vi "TOOLweb Spektren Pfad pruefen.vi"(6 "Aktionen":T3, 10 "labBaseName - SOLL":T1 caption="(82) labBaseName", 11 "Pfad Spektren - SOLL":T2 caption="Pfad Spektren") -> (2 "labBaseName - SOLL":T1 caption="(82) labBaseName", 3 "Pfad Spektren - SOLL":T2 caption="Pfad Spektren")   [LabVIEW 2020, in "FT-IR.lvlib" / "TOOLweb Interface.lvlib"]
doc: "Holt mit einer HTTP-POST-Anforderung gemäß TOOLweb-Protokoll Messdaten, Einstellungen und Diagnose-Information vom MKS MultiGas 2030 Analyzer. Alle Daten werden zeitsparend in einem einzigen Poll Request zusammengefasst, damit nur einmal eine TCP/IP-Verbindung geöffnet werden muss.\n\nAlle Ergebnis-Datentypen sind als Typdefinitionen in der Bibliothek \"Datentypen\" enthalten\" und erlauben so eine spätere Erweiterung.\n\nFalls \"Anzahl Gase\" unverbunden bleibt, wird der Standardwert 18 verwendet.\n \nFalls der TOOLWeb-Server nicht auf demselben Rechner arbeitet, kann mit \"IP-Adresse\" eine beliebiger Host adressiert werden. Ein unverbundener Eingang spricht den lokalen Host an."
uses:
  TOOLweb Interface.lvlib
  Spekten Pfad pruefen Aktionen.ctl
  Visualisierungs Elemente/Pfad-Eingabefeld.ctl
  Visualisierungs Elemente/String - Eingabefeld.ctl
  FGV FT-IR Aktionen.ctl
  FT-IR.lvlib
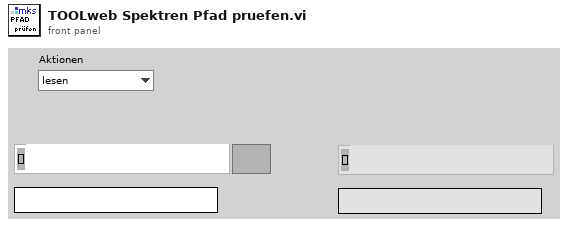
[diagram p1: front panel]
types:
  T1 = typedef "String - Eingabefeld.ctl" = string
  T2 = typedef "Pfad-Eingabefeld.ctl" = path
  T3 = typedef "FT-IR.lvlib/TOOLweb Interface.lvlib/Spekten Pfad pruefen Aktionen.ctl" = enum16{"lesen", "init", "prüfen", "setzen"}
  T4 = typedef "FT-IR.lvlib/FGV FT-IR Aktionen.ctl" = enum16{"lesen", "NOG setzen", "NOS setzen", "Initialisieren", "speichern", "ALLES setzen", "FT-IR Spektrum loggen", "Komm Stoppen", "Spektrum LogKonfig"}
  T5 = cluster{"(80) labEnabled":bool, "(81) labPath":path, "(82) labBaseName":string, "(83) labIndex":string, "Spektrum loggen aktiv?":bool}
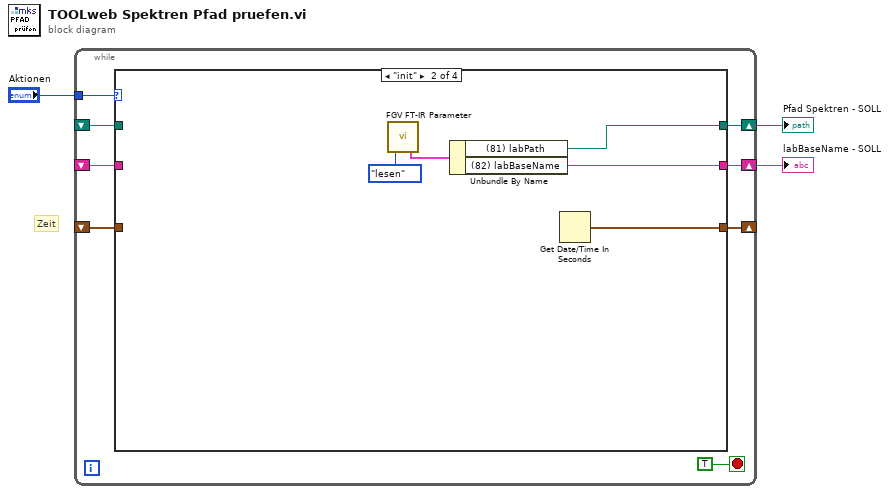
[diagram p0: block diagram]
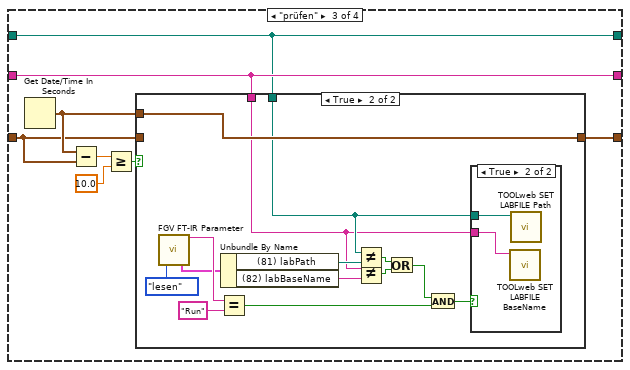
[diagram p3: hidden frame]
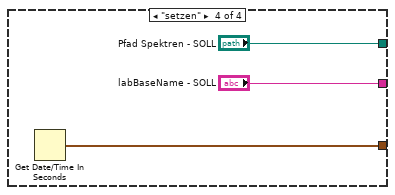
[diagram p6: hidden frame]
diagram:
  # "Zeit"
  n1 = while {
    shift-right: [w8] -> w2
    shift-left: _ -> [w6]
    shift-right: [w7] -> w1
    shift-left: _ -> [w5]
    tunnel: "Aktionen" -> [w10]
    shift-right: [w9] -> _
    shift-left: _ -> [w4]
    stop <- TRUE stop-if-true
    n2 = case shown="\"init\"" w10 {
      tunnel: [w12 w19 w23 w47] -> w9
      tunnel: [w14 w17 w20 "Pfad Spektren - SOLL"] -> w8
      tunnel: [w13 w16 w21 "labBaseName - SOLL"] -> w7
      tunnel: w6 -> [w14 _ w20 _]
      tunnel: w5 -> [w13 _ w21 _]
      tunnel: w4 -> [w12 _ w22 _]
      frame "lesen", Default {
      }
      frame "init" {
        n3 = call "FGV FT-IR Parameter.vi"("Aktion"=FGV_FT-IR_Aktionen."lesen") -> ("Ausgangs-Cluster"=w18:T5)  [unwired: 11 in, 7 out]
        n4 = Unbundle By Name(w18) -> ("(81) labPath"=w17:path, "(82) labBaseName"=w16:string)
        n5 = Get Date/Time In Seconds() -> (seconds since 1Jan1904=w19:timestamp)
      }
      frame "prüfen" {
        n6 = Get Date/Time In Seconds() -> (seconds since 1Jan1904=w24:timestamp)
        n7 = Subtract(x=w24, y=w22) -> (x-y=w26:dbl)
        n8 = Greater Or Equal?(x=w26, y=10.0) -> (x >= y?=w25:bool)
        n9 = case shown="True" w25 {
          tunnel: w24 -> [_ w42]
          tunnel: [w28 w42] -> w23
          tunnel: w22 -> [w28 _]
          tunnel: w21 -> [_ w30]
          tunnel: w20 -> [_ w31]
          frame False {
          }
          frame True {
            n10 = call "FGV FT-IR Parameter.vi"("Aktion"=FGV_FT-IR_Aktionen."lesen") -> ("Ausgangs-Cluster"=w38:T5, "Instrument State"=w39:string)  [unwired: 11 in, 6 out]
            n11 = Equal?(x=w39, y="Run") -> (x = y?=w32:bool)
            n12 = Unbundle By Name(w38) -> ("(81) labPath"=w37:path, "(82) labBaseName"=w36:string)
            n13 = Not Equal?(x=w31, y=w37) -> (x != y?=w35:bool)
            n14 = Not Equal?(x=w30, y=w36) -> (x != y?=w34:bool)
            n15 = Or(x=w35, y=w34) -> (x .or. y?=w33:bool)
            n16 = And(x=w33, y=w32) -> (x .and. y?=w29:bool)
            n17 = case shown="True" w29 {
              tunnel: w31 -> [_ w44]
              tunnel: w30 -> [_ w43]
              frame False {
              }
              frame True {
                n18 = call "TOOLweb SET LABFILE BaseName.vi"("BaseName"=w43) -> ()  [unwired: 2 in, 5 out]
                n19 = call "TOOLweb SET LABFILE Path.vi"("labPath"=w44) -> ()  [unwired: 2 in, 5 out]
              }
            }
          }
        }
      }
      frame "setzen" {
        n20 = Get Date/Time In Seconds() -> (seconds since 1Jan1904=w47:timestamp)
      }
    }
  }
  "Pfad Spektren - SOLL" <- w2
  "labBaseName - SOLL" <- w1
